vi "DCMCT_Position_Digital_Scopes.vi"(1 "Position (rad)":dbl, 2 "Speed (rad/s)":dbl, 3 "Current (A)":dbl) -> (0 "Digital Scopes":T1)   [LabVIEW 2011]
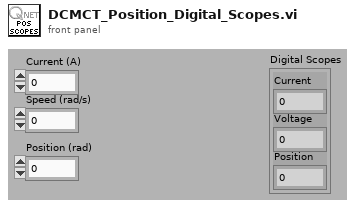
[diagram p1: front panel]
types:
  T1 = cluster{"Current":dbl, "Voltage":dbl, "Position":dbl}
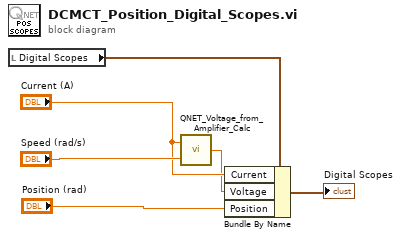
[diagram p0: block diagram]
diagram:
  n1 = local read "Digital Scopes"() -> (w2:T1)
  n2 = call "QNET_Voltage_from_Amplifier_Calc.vi"("Speed (rad/s)"="Speed (rad/s)", "Im (A)"="Current (A)") -> ("Vm (V)"=w4:dbl)
  n3 = Bundle By Name(cluster=w2, "Current"="Current (A)", "Voltage"=w4, "Position"="Position (rad)") -> (→"Digital Scopes":T1)
